vi "Get Fit Results String.vi"(7 "Plot Name":string, 8 "error in (no error)":errorcluster, 9 "Fit Parameters Uncertainties Cluster":variant, 10 "Fit Model":T1, 11 "Fit Parameters Cluster":variant) -> (0 "error out":errorcluster, 3 "Fit Results String":string)   [LabVIEW 2019]
uses:
  Fit Models.ctl
  Gaussian/Gaussian Fit Results v2.ctl
  Lorentzian/Lorentzian Fit Results v2.ctl
  Asymmetric Gaussian/Asymmetric Gaussian Fit Results v2.ctl
  Asymmetric Lorentzian/Asymmetric Lorentzian Fit Results v2.ctl
  Gaussian-Lorentzian/Gaussian-Lorentzian Fit Results v2.ctl
  Lorentzian-Gaussian/Lorentzian-Gaussian Fit Results v2.ctl
  Two Connected Gaussians/Two H-Connected Gaussians Fit Parameters.ctl
  Two Connected Gaussians/Two T-Connected Gaussians Fit Parameters.ctl
  Two Connected Asymmetric Gaussians/Two T-Connected Asymmetric Gaussians Fit Parameters.ctl
  Two Connected Asymmetric Gaussians/Two H-Connected Asymmetric Gaussians Fit Parameters.ctl
  Single Exponential/Single Exponential Fit Parameters v2.ctl
  IRF(X)PSED/IRF(X)PSED Fit Parameters.ctl
  Double Exponential/Double Exponential Fit Parameters v2.ctl
  ACF-CCF/2D ACF/2D Gaussian ACF Fit Results.ctl
  ACF-CCF/2D ACF/2D Gaussian + Blinking ACF Fit Results.ctl
  ACF-CCF/2D ACF/2D Gaussian + Flow ACF Fit Results.ctl
  ACF-CCF/3D ACF/3D Gaussian ACF Fit Results.ctl
  ACF-CCF/3D ACF/3D Gaussian + Blinking ACF Fit Results.ctl
  ACF-CCF/2D ACF/2D Gaussian ACF & 2D Gaussian ACF + Flow Fit Results.ctl
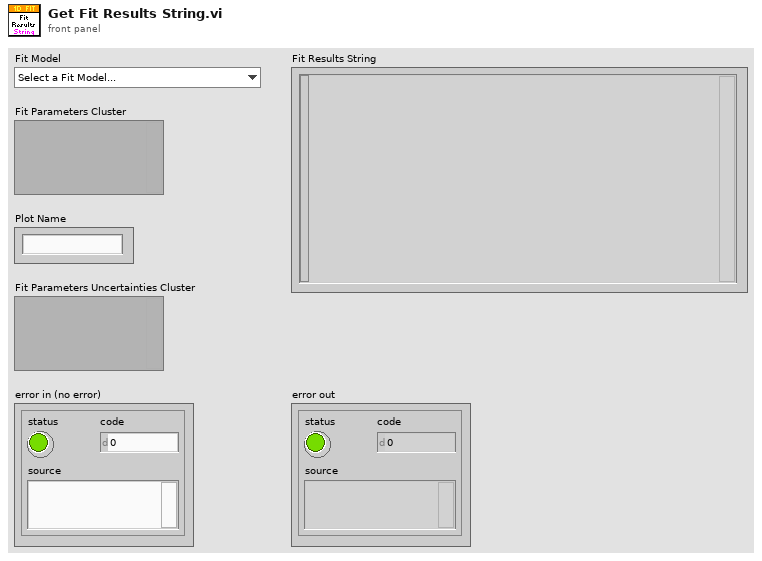
[diagram p1: front panel]
types:
  T1 = typedef "Fit Models.ctl" = enum16{"Select a Fit Model...", "           Single Peak", "Gaussian", "Asymmetric Gaussian", "Lorentzian", "Asymmetric Lorentzian", "Gaussian/Lorentzian", "Lorentzian/Gaussian", "           Double Peak", "Two Gaussians", "Two Asymmetric Gaussians", "Two H-Connected Gaussians", "Two T-Connected Gaussians", "Two H-Connected Asymmetric Gaussians", "Two T-Connected Asymmetric Gaussians", "           Triple Peak", "Three Gaussians", "Three Asymmetric Gaussians", "              Decays", "1-Exponential", "IRF*PSED", "2-Exponentials", "               ACF", "2D Gaussian ACF", "2D Gaussian + Blinking ACF", "2D Gaussian + Flow ACF", "3D Gaussian ACF", "3D Gaussian + Blinking ACF", "             Multiplot", "2D Gaussian ACF & 2D Gaussian + Flow ACF"}
  T2 = typedef "Gaussian Fit Results v2.ctl" = cluster{"Amplitude":dbl, "Peak":dbl, "SDV":dbl, "FWHM":dbl, "Integral":dbl, "RMSE":dbl, "R^2":dbl}
  T3 = typedef "Lorentzian Fit Results v2.ctl" = cluster{"Amplitude":dbl, "Peak":dbl, "FWHM":dbl, "Integral":dbl, "RMSE":dbl, "R^2":dbl}
  T4 = typedef "Asymmetric Gaussian Fit Results v2.ctl" = cluster{"Amplitude":dbl, "Peak":dbl, "SDV-":dbl, "SDV+":dbl, "Mean":dbl, "SDV":dbl, "FWHM":dbl, "Integral":dbl, "RMSE":dbl, "R^2":dbl}
  T5 = typedef "Asymmetric Lorentzian Fit Results v2.ctl" = cluster{"Amplitude":dbl, "Peak":dbl, "FWHM-":dbl, "FWHM+":dbl, "Integral":dbl, "RMSE":dbl, "R^2":dbl}
  T6 = typedef "Gaussian-Lorentzian Fit Results v2.ctl" = cluster{"Amplitude":dbl, "Peak":dbl, "SDV-":dbl, "FWHM+":dbl, "Mean":dbl, "FWHM":dbl, "Integral":dbl, " RMSE":dbl, "R^2":dbl}
  T7 = typedef "Lorentzian-Gaussian Fit Results v2.ctl" = cluster{"Amplitude":dbl, "Peak":dbl, "FWHM-":dbl, "SDV+":dbl, "Mean":dbl, "FWHM":dbl, "Integral":dbl, "RMSE":dbl, "R^2":dbl}
  T8 = typedef "Two H-Connected Gaussians Fit Parameters.ctl" = cluster{"Gaussian Parameters":T2[], "Bridge Amplitude ":dbl}
  T9 = typedef "Two T-Connected Gaussians Fit Parameters.ctl" = cluster{"Gaussian Parameters":T2[], "Bridge Amplitude ":dbl, "Bridge Slope":dbl}
  T10 = typedef "Two T-Connected Asymmetric Gaussians Fit Parameters.ctl" = cluster{"Asymmetric Gaussian Parameters":T4[], "Bridge Amplitude":dbl, "Bridge Slope":dbl}
  T11 = typedef "Two H-Connected Asymmetric Gaussians Fit Parameters.ctl" = cluster{"Asymmetric Gaussian Parameters":T4[], "Bridge Amplitude":dbl}
  T12 = typedef "Single Exponential Fit Parameters v2.ctl" = cluster{"Amplitude":dbl, "Time Constant":dbl, "Baseline":dbl, "Mean":dbl, "SDV":dbl, "FWHM":dbl, "Integral":dbl, "MSE":dbl, "R^2":dbl}
  T13 = typedef "IRF(X)PSED Fit Parameters.ctl" = cluster{"Offset":dbl, "Amplitudes":dbl[], "Time Constants":dbl[], "Baseline":dbl, "Lifetime":dbl, "IRF order":dbl, "Period":dbl, "SDV":dbl, "FWHM":dbl, "Integral":dbl, "MSE":dbl, "R^2":dbl}
  T14 = typedef "Double Exponential Fit Parameters v2.ctl" = cluster{"A1":dbl, "tau1":dbl, "A2":dbl, "tau2":dbl, "Baseline":dbl, "Mean":dbl, "SDV":dbl, "Integral":dbl, "MSE":dbl, "R^2":dbl}
  T15 = typedef "2D Gaussian ACF Fit Results.ctl" = cluster{"Amplitude":dbl, "Diffusion Time":dbl, "RMSE":dbl, "R^2":dbl}
  T16 = typedef "2D Gaussian + Blinking ACF Fit Results.ctl" = cluster{"Amplitude":dbl, "Diffusion Time":dbl, "Blinking Fraction":dbl, "Blinking Time Constant":dbl, "RMSE":dbl, "R^2":dbl}
  T17 = typedef "2D Gaussian + Flow ACF Fit Results.ctl" = cluster{"Amplitude":dbl, "Diffusion Time":dbl, "Translation Time":dbl, "RMSE":dbl, "R^2":dbl}
  T18 = typedef "3D Gaussian ACF Fit Results.ctl" = cluster{"Amplitude":dbl, "Diffusion Time":dbl, "Aspect Ratio":dbl, "RMSE":dbl, "R^2":dbl}
  T19 = typedef "3D Gaussian + Blinking ACF Fit Results.ctl" = cluster{"Amplitude":dbl, "Diffusion Time":dbl, "Aspect Ratio":dbl, "Blinking Fraction":dbl, "Blinking Time Constant":dbl, "RMSE":dbl, "R^2":dbl}
  T20 = typedef "2D Gaussian ACF & 2D Gaussian ACF + Flow Fit Results.ctl" = cluster{"Amplitude 1":dbl, "Diffusion Time":dbl, "Amplitude 2":dbl, "Translation Time":dbl, "RMSE":dbl, "R^2":dbl}
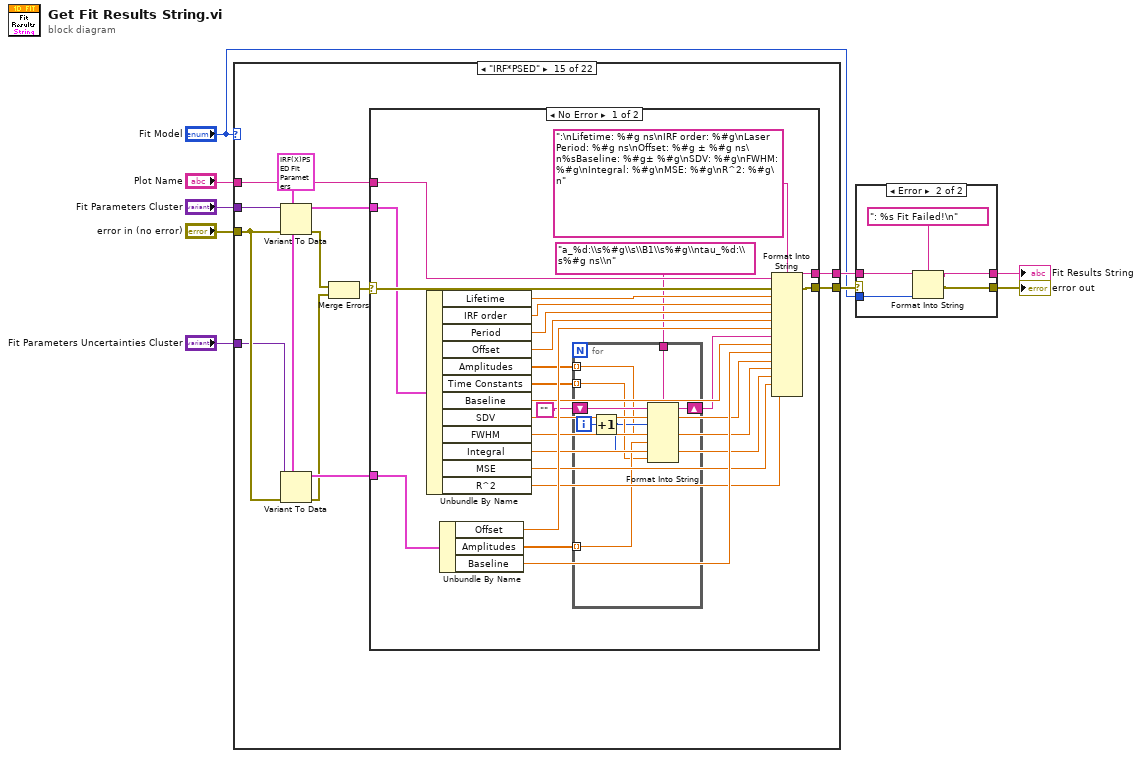
[diagram p0: block diagram]
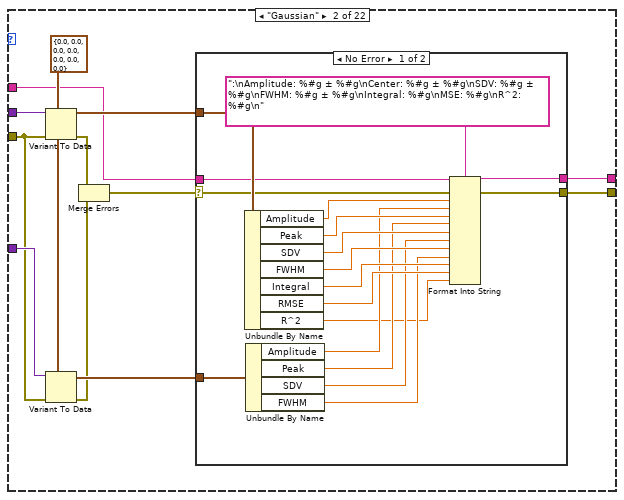
[diagram p4: hidden frame]
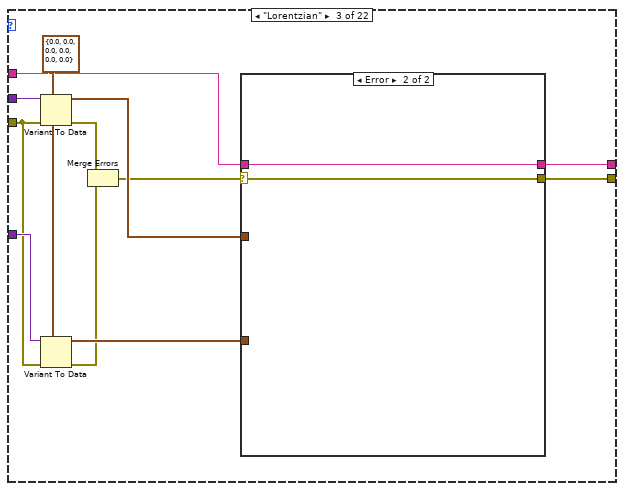
[diagram p6: hidden frame]
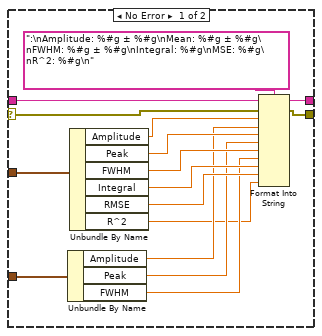
[diagram p7: hidden frame]
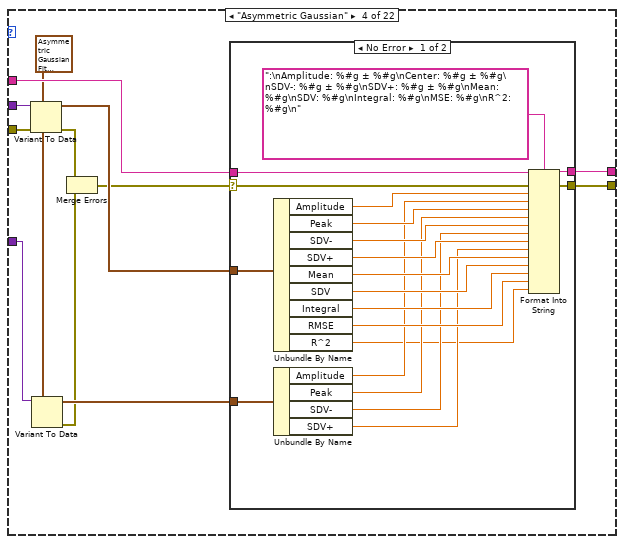
[diagram p8: hidden frame]
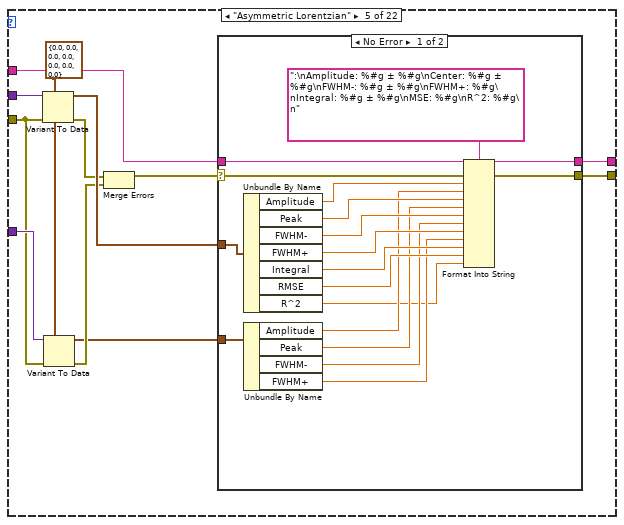
[diagram p10: hidden frame]
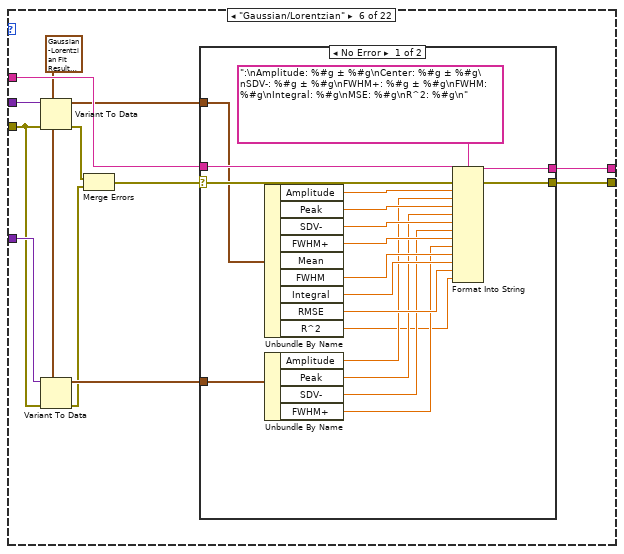
[diagram p12: hidden frame]
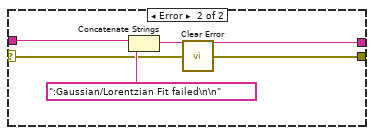
[diagram p13: hidden frame]
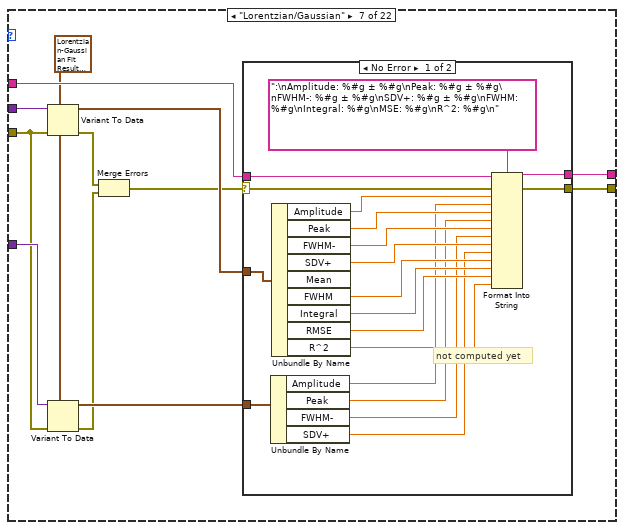
[diagram p14: hidden frame]
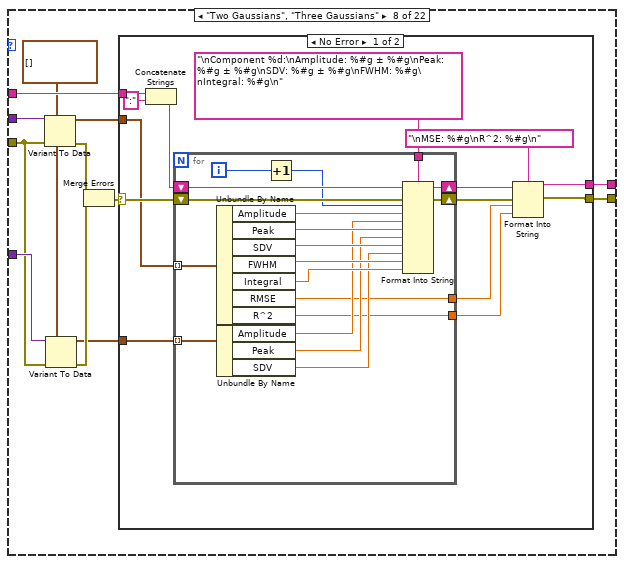
[diagram p16: hidden frame]
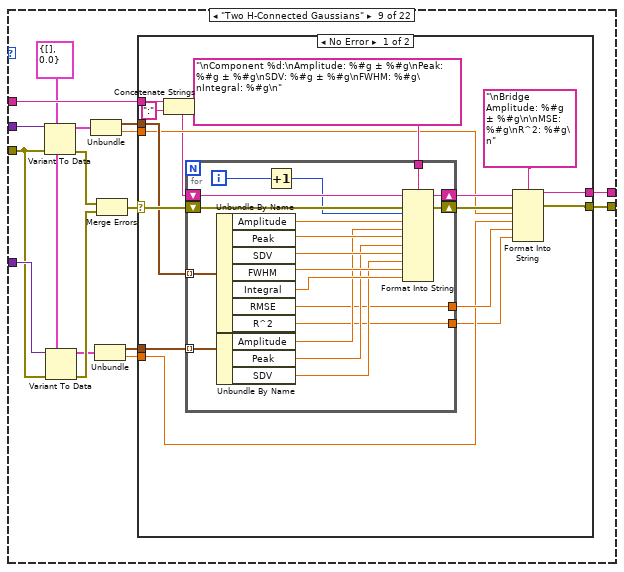
[diagram p18: hidden frame]
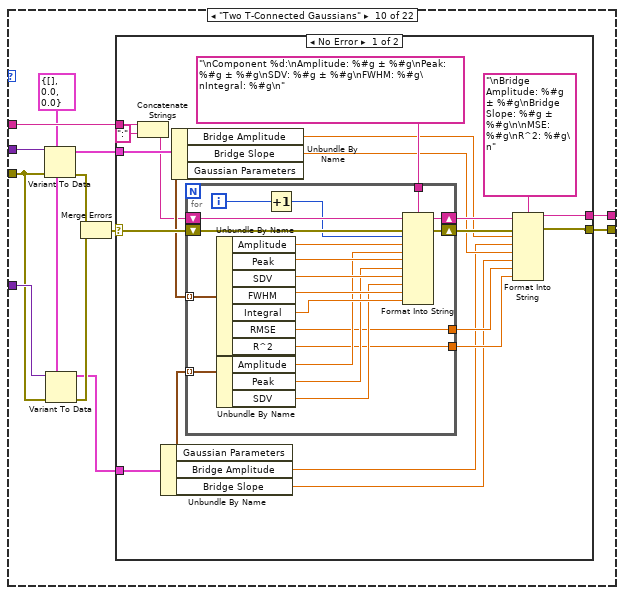
[diagram p20: hidden frame]
diagram:
  n1 = case shown="\"IRF*PSED\"" "Fit Model" {
    tunnel: "error in (no error)" -> [w10 w15 w46 w81 w110 w141 w175 w214 w265 w314 w366 w417 w474 w531 w564 w611 w644 w671 w702 w731 w761 w794]
    tunnel: [w10 w22 w53 w83 w118 w149 w185 w218 w269 w318 w371 w422 w479 w534 w567 w614 w651 w678 w709 w738 w767 w800] -> w5
    tunnel: [_ w21 w54 w84 w117 w150 w186 w219 w270 w319 w372 w423 w480 w535 w568 w615 w650 w677 w708 w737 w766 w799] -> w3
    tunnel: "Fit Parameters Cluster" -> [_ w20 w52 w82 w115 w147 w183 w216 w267 w316 w369 w420 w477 w530 w563 w613 w649 w676 w707 w736 w765 w798]
    tunnel: "Fit Parameters Uncertainties Cluster" -> [_ w18 w50 w76 w111 w142 w179 w215 w266 w315 w367 w418 w475 w524 w557 w612 w647 w674 w705 w734 w763 w796]
    tunnel: "Plot Name" -> [_ w11 w47 w80 w116 w148 w184 w217 w268 w317 w370 w421 w478 w525 w558 w604 w640 w667 w698 w727 w757 w790]
    frame "Select a Fit Model...", Default {
    }
    frame "Gaussian" {
      w17 = T2 {"Amplitude"=0.0, "Peak"=0.0, "SDV"=0.0, "FWHM"=0.0, "Integral"=0.0, "RMSE"=0.0, "R^2"=0.0} ("Gaussian Fit Parameters")
      n2 = Variant To Data(error in=w15, type=w17, Variant=w20) -> (data=w19:T2, error out=w14:errorcluster)
      n3 = Variant To Data(error in=w15, type=w17, Variant=w18) -> (data=w16:T2, error out=w13:errorcluster)
      n4 = Merge Errors(w14, w13) -> (w12:errorcluster)
      n5 = case shown="No Error" w12 {
        selector: w12 -> [w30 w41]
        tunnel: [w40 w41] -> w22
        tunnel: [w39 w42] -> w21
        tunnel: w11 -> [w24 w42]
        tunnel: w19 -> [w37 _]
        tunnel: w16 -> [w29 _]
        frame No Error {
          n6 = Unbundle By Name(w37) -> ("Amplitude"=w36:dbl, "Peak"=w35:dbl, "SDV"=w34:dbl, "FWHM"=w32:dbl, "Integral"=w33:dbl, "RMSE"=w31:dbl, "R^2"=w23:dbl)
          n7 = Unbundle By Name(w29) -> ("Amplitude"=w28:dbl, "Peak"=w27:dbl, "SDV"=w26:dbl, "FWHM"=w25:dbl)
          n8 = Format Into String(format string=":\nAmplitude: %#g ± %#g\nCenter: %#g ± %#g\nSDV: %#g ± %#g\nFWHM: %#g ± %#g\nIntegral: %#g\nMSE: %#g\nR^2: %#g\n", initial string=w24, error in=w30, w36, w28, w35, w27, w34, w26, w32, w25, w33, w31, w23) -> (resulting string=w39:string, error out=w40:errorcluster)
        }
        frame Error {
        }
      }
    }
    frame "Lorentzian" {
      w48 = T3 {"Amplitude"=0.0, "Peak"=0.0, "FWHM"=0.0, "Integral"=0.0, "RMSE"=0.0, "R^2"=0.0} ("Lorentz Fit Parameters")
      n9 = Variant To Data(error in=w46, type=w48, Variant=w52) -> (data=w51:T3, error out=w45:errorcluster)
      n10 = Variant To Data(error in=w46, type=w48, Variant=w50) -> (data=w49:T3, error out=w44:errorcluster)
      n11 = Merge Errors(w45, w44) -> (w43:errorcluster)
      n12 = case shown="Error" w43 {
        selector: w43 -> [w61 w71]
        tunnel: w47 -> [w70 w72]
        tunnel: w51 -> [w69 _]
        tunnel: [w63 w72] -> w54
        tunnel: [w62 w71] -> w53
        tunnel: w49 -> [w59 _]
        frame No Error {
          n13 = Unbundle By Name(w59) -> ("Amplitude"=w58:dbl, "Peak"=w57:dbl, "FWHM"=w56:dbl)
          n14 = Unbundle By Name(w69) -> ("Amplitude"=w67:dbl, "Peak"=w68:dbl, "FWHM"=w66:dbl, "Integral"=w65:dbl, "RMSE"=w64:dbl, "R^2"=w55:dbl)
          n15 = Format Into String(format string=":\nAmplitude: %#g ± %#g\nMean: %#g ± %#g\nFWHM: %#g ± %#g\nIntegral: %#g\nMSE: %#g\nR^2: %#g\n", initial string=w70, error in=w61, w67, w58, w68, w57, w66, w56, w65, w64, w55) -> (resulting string=w63:string, error out=w62:errorcluster)
        }
        frame Error {
        }
      }
    }
    frame "Asymmetric Gaussian" {
      w78 = T4 {"Amplitude"=0.0, "Peak"=0.0, "SDV-"=0.0, "SDV+"=0.0, "Mean"=0.0, "SDV"=0.0, "FWHM"=0.0, "Integral"=0.0, "RMSE"=0.0, "R^2"=0.0} ("Asymmetric Gaussian Fit Parameters")
      n16 = Variant To Data(error in=w81, type=w78, Variant=w82) -> (data=w79:T4, error out=w75:errorcluster)
      n17 = Variant To Data(type=w78, Variant=w76) -> (data=w77:T4, error out=w74:errorcluster)  [unwired: 1 in]
      n18 = Merge Errors(w75, w74) -> (w73:errorcluster)
      n19 = case shown="No Error" w73 {
        selector: w73 -> [w102 w106]
        tunnel: w80 -> [w104 w105]
        tunnel: w79 -> [w91 _]
        tunnel: [w93 w105] -> w84
        tunnel: [w92 w106] -> w83
        tunnel: w77 -> [w90 _]
        frame No Error {
          n20 = Unbundle By Name(w91) -> ("Amplitude"=w98:dbl, "Peak"=w101:dbl, "SDV-"=w100:dbl, "SDV+"=w99:dbl, "Mean"=w97:dbl, "SDV"=w96:dbl, "Integral"=w95:dbl, "RMSE"=w94:dbl, "R^2"=w85:dbl)
          n21 = Unbundle By Name(w90) -> ("Amplitude"=w89:dbl, "Peak"=w88:dbl, "SDV-"=w87:dbl, "SDV+"=w86:dbl)
          n22 = Format Into String(format string=":\nAmplitude: %#g ± %#g\nCenter: %#g ± %#g\nSDV-: %#g ± %#g\nSDV+: %#g ± %#g\nMean: %#g\nSDV: %#g\nIntegral: %#g\nMSE: %#g\nR^2: %#g\n", initial string=w104, error in=w102, w98, w89, w101, w88, w100, w87, w99, w86, w97, w96, w95, w94, w85) -> (resulting string=w93:string, error out=w92:errorcluster)
        }
        frame Error {
        }
      }
    }
    frame "Asymmetric Lorentzian" {
      w112 = T5 {"Amplitude"=0.0, "Peak"=0.0, "FWHM-"=0.0, "FWHM+"=0.0, "Integral"=0.0, "RMSE"=0.0, "R^2"=0.0} ("Asymmetric Lorentz Fit Parameters")
      n23 = Variant To Data(error in=w110, type=w112, Variant=w115) -> (data=w114:T5, error out=w113:errorcluster)
      n24 = Variant To Data(error in=w110, type=w112, Variant=w111) -> (data=w108:T5, error out=w109:errorcluster)
      n25 = Merge Errors(w113, w109) -> (w107:errorcluster)
      n26 = case shown="No Error" w107 {
        selector: w107 -> [w135 w138]
        tunnel: [w128 w138] -> w118
        tunnel: [w127 w137] -> w117
        tunnel: w116 -> [w122 w137]
        tunnel: w114 -> [w121 _]
        tunnel: w108 -> [w120 _]
        frame No Error {
          n27 = Unbundle By Name(w121) -> ("Amplitude"=w131:dbl, "Peak"=w134:dbl, "FWHM-"=w133:dbl, "FWHM+"=w132:dbl, "Integral"=w130:dbl, "RMSE"=w129:dbl, "R^2"=w119:dbl)
          n28 = Unbundle By Name(w120) -> ("Amplitude"=w126:dbl, "Peak"=w125:dbl, "FWHM-"=w124:dbl, "FWHM+"=w123:dbl)
          n29 = Format Into String(format string=":\nAmplitude: %#g ± %#g\nCenter: %#g ± %#g\nFWHM-: %#g ± %#g\nFWHM+: %#g\nIntegral: %#g ± %#g\nMSE: %#g\nR^2: %#g\n", initial string=w122, error in=w135, w131, w126, w134, w125, w133, w124, w132, w123, w130, w129, w119) -> (resulting string=w127:string, error out=w128:errorcluster)
        }
        frame Error {
        }
      }
    }
    frame "Gaussian/Lorentzian" {
      w143 = T6 {"Amplitude"=0.0, "Peak"=0.0, "SDV-"=0.0, "FWHM+"=0.0, "Mean"=0.0, "FWHM"=0.0, "Integral"=0.0, " RMSE"=0.0, "R^2"=0.0} ("Gaussian/Lorentzian Fit Parameters")
      n30 = Variant To Data(error in=w141, type=w143, Variant=w147) -> (data=w144:T6, error out=w146:errorcluster)
      n31 = Variant To Data(error in=w141, type=w143, Variant=w142) -> (data=w140:T6, error out=w139:errorcluster)
      n32 = Merge Errors(w146, w139) -> (w145:errorcluster)
      n33 = case shown="No Error" w145 {
        selector: w145 -> [w167 w171]
        tunnel: w148 -> [w169 w173]
        tunnel: [w159 w172] -> w150
        tunnel: [w158 w170] -> w149
        tunnel: w144 -> [w153 _]
        tunnel: w140 -> [w152 _]
        frame No Error {
          n34 = Unbundle By Name(w153) -> ("Amplitude"=w165:dbl, "Peak"=w166:dbl, "SDV-"=w164:dbl, "FWHM+"=w163:dbl, "FWHM"=w162:dbl, "Integral"=w161:dbl, "RMSE"=w160:dbl, "R^2"=w151:dbl)  [unwired: 1 out]
          n35 = Unbundle By Name(w152) -> ("Amplitude"=w157:dbl, "Peak"=w156:dbl, "SDV-"=w155:dbl, "FWHM+"=w154:dbl)
          n36 = Format Into String(format string=":\nAmplitude: %#g ± %#g\nCenter: %#g ± %#g\nSDV-: %#g ± %#g\nFWHM+: %#g ± %#g\nFWHM: %#g\nIntegral: %#g\nMSE: %#g\nR^2: %#g\n", initial string=w169, error in=w167, w165, w157, w166, w156, w164, w155, w163, w154, w162, w161, w160, w151) -> (resulting string=w159:string, error out=w158:errorcluster)
        }
        frame Error {
          n37 = Concatenate Strings(w173, ":Gaussian/Lorentzian Fit failed\n\n" ("format string")) -> (w172:string)
          n38 = call "Clear Error.vi"("Error In"=w171) -> ("no Error Out"=w170:errorcluster)  [unwired: 8 in]
        }
      }
    }
    frame "Lorentzian/Gaussian" {
      w178 = T7 {"Amplitude"=0.0, "Peak"=0.0, "FWHM-"=0.0, "SDV+"=0.0, "Mean"=0.0, "FWHM"=0.0, "Integral"=0.0, "RMSE"=0.0, "R^2"=0.0} ("Lorentzian/Gaussian Fit Parameters")
      n39 = Variant To Data(error in=w175, type=w178, Variant=w183) -> (data=w182:T7, error out=w181:errorcluster)
      n40 = Variant To Data(error in=w175, type=w178, Variant=w179) -> (data=w177:T7, error out=w176:errorcluster)
      n41 = Merge Errors(w181, w176) -> (w180:errorcluster)
      n42 = case shown="No Error" w180 {
        selector: w180 -> [w204 w207]
        tunnel: [w196 w206] -> w186
        tunnel: [w195 w207] -> w185
        tunnel: w184 -> [w190 w206]
        tunnel: w182 -> [w189 _]
        tunnel: w177 -> [w188 _]
        frame No Error {
          # "not computed yet"
          n43 = Unbundle By Name(w188) -> ("Amplitude"=w194:dbl, "Peak"=w193:dbl, "FWHM-"=w192:dbl, "SDV+"=w191:dbl)
          n44 = Unbundle By Name(w189) -> ("Amplitude"=w202:dbl, "Peak"=w203:dbl, "FWHM-"=w200:dbl, "SDV+"=w201:dbl, "FWHM"=w199:dbl, "Integral"=w198:dbl, "RMSE"=w197:dbl, "R^2"=w187:dbl)  [unwired: 1 out]
          n45 = Format Into String(format string=":\nAmplitude: %#g ± %#g\nPeak: %#g ± %#g\nFWHM-: %#g ± %#g\nSDV+: %#g ± %#g\nFWHM: %#g\nIntegral: %#g\nMSE: %#g\nR^2: %#g\n", initial string=w190, error in=w204, w202, w194, w203, w193, w200, w192, w201, w191, w199, w198, w197, w187) -> (resulting string=w196:string, error out=w195:errorcluster)
        }
        frame Error {
        }
      }
    }
    frame "Two Gaussians", "Three Gaussians" {
      w208 = T2[] [] ("Array")
      n46 = Variant To Data(error in=w214, type=w208, Variant=w216) -> (data=w210:T2[], error out=w213:errorcluster)
      n47 = Variant To Data(error in=w214, type=w208, Variant=w215) -> (data=w209:T2[], error out=w212:errorcluster)
      n48 = Merge Errors(w213, w212) -> (w211:errorcluster)
      n49 = case shown="No Error" w211 {
        selector: w211 -> [w232 w254]
        tunnel: [w227 w253] -> w219
        tunnel: [w225 w254] -> w218
        tunnel: w217 -> [w230 w253]
        tunnel: w210 -> [w229 _]
        tunnel: w209 -> [w228 _]
        frame No Error {
          n50 = Concatenate Strings(w230, ":" ("string")) -> (w221:string)
          n51 = for {
            tunnel: "\nComponent %d:\nAmplitude: %#g ± %#g\nPeak: %#g ± %#g\nSDV: %#g ± %#g\nFWHM: %#g\nIntegral: %#g\n" ("format string") -> [w252]
            shift-right: [w245] -> w226
            shift-left: w232 -> [w251]
            shift-right: [w246] -> w231
            shift-left: w221 -> [w244]
            tunnel: w229 -> [w237] mode=indexing
            tunnel: w228 -> [w236] mode=indexing
            tunnel: [w235] -> w223
            tunnel: [w234] -> w222
            i -> [w239]
            n52 = Unbundle By Name(w237) -> ("Amplitude"=w240:dbl, "Peak"=w250:dbl, "SDV"=w249:dbl, "FWHM"=w248:dbl, "Integral"=w247:dbl, "RMSE"=w235:dbl, "R^2"=w234:dbl)
            n53 = Unbundle By Name(w236) -> ("Amplitude"=w243:dbl, "Peak"=w242:dbl, "SDV"=w241:dbl)
            n54 = Increment(x=w239) -> (x+1=w238:i32)
            n55 = Format Into String(format string=w252, initial string=w244, error in=w251, w238, w240, w243, w250, w242, w249, w241, w248, w247) -> (resulting string=w246:string, error out=w245:errorcluster)
          }
          n56 = Format Into String(format string="\nMSE: %#g\nR^2: %#g\n", initial string=w231, error in=w226, w223, w222) -> (resulting string=w227:string, error out=w225:errorcluster)
        }
        frame Error {
        }
      }
    }
    frame "Two H-Connected Gaussians" {
      w259 = T8 {"Gaussian Parameters"=[], "Bridge Amplitude "=0.0} ("Bridged Gaussians Parameters")
      n57 = Variant To Data(error in=w265, type=w259, Variant=w267) -> (data=w261:T8, error out=w264:errorcluster)
      n58 = Variant To Data(error in=w265, type=w259, Variant=w266) -> (data=w260:T8, error out=w263:errorcluster)
      n59 = Unbundle(w261) -> ("Gaussian Parameters"=w258:T2[], "Bridge Amplitude"=w256:dbl)
      n60 = Unbundle(w260) -> ("Gaussian Parameters"=w257:T2[], "Bridge Amplitude"=w255:dbl)
      n61 = Merge Errors(w264, w263) -> (w262:errorcluster)
      n62 = case shown="No Error" w262 {
        selector: w262 -> [w285 w307]
        tunnel: [w281 w306] -> w270
        tunnel: [w279 w307] -> w269
        tunnel: w268 -> [w272 w306]
        tunnel: w258 -> [w283 _]
        tunnel: w257 -> [w282 _]
        tunnel: w256 -> [w275 _]
        tunnel: w255 -> [w276 _]
        frame No Error {
          n63 = Concatenate Strings(w272, ":" ("string")) -> (w271:string)
          n64 = for {
            tunnel: "\nComponent %d:\nAmplitude: %#g ± %#g\nPeak: %#g ± %#g\nSDV: %#g ± %#g\nFWHM: %#g\nIntegral: %#g\n" ("format string") -> [w305]
            shift-right: [w298] -> w280
            shift-left: w285 -> [w304]
            shift-right: [w299] -> w284
            shift-left: w271 -> [w297]
            tunnel: w283 -> [w290] mode=indexing
            tunnel: w282 -> [w289] mode=indexing
            tunnel: [w288] -> w277
            tunnel: [w287] -> w274
            i -> [w292]
            n65 = Unbundle By Name(w290) -> ("Amplitude"=w293:dbl, "Peak"=w303:dbl, "SDV"=w302:dbl, "FWHM"=w301:dbl, "Integral"=w300:dbl, "RMSE"=w288:dbl, "R^2"=w287:dbl)
            n66 = Unbundle By Name(w289) -> ("Amplitude"=w296:dbl, "Peak"=w295:dbl, "SDV"=w294:dbl)
            n67 = Increment(x=w292) -> (x+1=w291:i32)
            n68 = Format Into String(format string=w305, initial string=w297, error in=w304, w291, w293, w296, w303, w295, w302, w294, w301, w300) -> (resulting string=w299:string, error out=w298:errorcluster)
          }
          n69 = Format Into String(format string="\nBridge Amplitude: %#g ± %#g\n\nMSE: %#g\nR^2: %#g\n", initial string=w284, error in=w280, w275, w276, w277, w274) -> (resulting string=w281:string, error out=w279:errorcluster)
        }
        frame Error {
        }
      }
    }
    frame "Two T-Connected Gaussians" {
      w310 = T9 {"Gaussian Parameters"=[], "Bridge Amplitude "=0.0, "Bridge Slope"=0.0} ("Bridged Gaussians Parameters")
      n70 = Variant To Data(error in=w314, type=w310, Variant=w316) -> (data=w309:T9, error out=w313:errorcluster)
      n71 = Variant To Data(error in=w314, type=w310, Variant=w315) -> (data=w308:T9, error out=w312:errorcluster)
      n72 = Merge Errors(w313, w312) -> (w311:errorcluster)
      n73 = case shown="No Error" w311 {
        selector: w311 -> [w338 w360]
        tunnel: [w336 w359] -> w319
        tunnel: [w334 w360] -> w318
        tunnel: w317 -> [w321 w359]
        tunnel: w309 -> [w330 _]
        tunnel: w308 -> [w326 _]
        frame No Error {
          n74 = Concatenate Strings(w321, ":" ("string")) -> (w320:string)
          n75 = Unbundle By Name(w326) -> ("Gaussian Parameters"=w325:T2[], "Bridge Amplitude"=w324:dbl, "Bridge Slope"=w323:dbl)
          n76 = Unbundle By Name(w330) -> ("Bridge Amplitude"=w328:dbl, "Bridge Slope"=w327:dbl, "Gaussian Parameters"=w329:T2[])
          n77 = for {
            tunnel: "\nComponent %d:\nAmplitude: %#g ± %#g\nPeak: %#g ± %#g\nSDV: %#g ± %#g\nFWHM: %#g\nIntegral: %#g\n" ("format string") -> [w358]
            shift-right: [w351] -> w335
            shift-left: w338 -> [w357]
            shift-right: [w352] -> w337
            shift-left: w320 -> [w350]
            tunnel: w329 -> [w343] mode=indexing
            tunnel: w325 -> [w342] mode=indexing
            tunnel: [w341] -> w332
            tunnel: [w340] -> w331
            i -> [w345]
            n78 = Unbundle By Name(w343) -> ("Amplitude"=w346:dbl, "Peak"=w356:dbl, "SDV"=w355:dbl, "FWHM"=w354:dbl, "Integral"=w353:dbl, "RMSE"=w341:dbl, "R^2"=w340:dbl)
            n79 = Unbundle By Name(w342) -> ("Amplitude"=w349:dbl, "Peak"=w348:dbl, "SDV"=w347:dbl)
            n80 = Increment(x=w345) -> (x+1=w344:i32)
            n81 = Format Into String(format string=w358, initial string=w350, error in=w357, w344, w346, w349, w356, w348, w355, w347, w354, w353) -> (resulting string=w352:string, error out=w351:errorcluster)
          }
          n82 = Format Into String(format string="\nBridge Amplitude: %#g ± %#g\nBridge Slope: %#g ± %#g\n\nMSE: %#g\nR^2: %#g\n", initial string=w337, error in=w335, w328, w324, w327, w323, w332, w331) -> (resulting string=w336:string, error out=w334:errorcluster)
        }
        frame Error {
        }
      }
    }
    frame "Two Asymmetric Gaussians", "Three Asymmetric Gaussians" {
      w365 = T4[] [] ("Array")
      n83 = Variant To Data(error in=w366, type=w365, Variant=w367) -> (data=w361:T4[], error out=w364:errorcluster)
      n84 = Variant To Data(error in=w366, type=w365, Variant=w369) -> (data=w362:T4[], error out=w368:errorcluster)
      n85 = Merge Errors(w368, w364) -> (w363:errorcluster)
      n86 = case shown="No Error" w363 {
        selector: w363 -> [w385 w410]
        tunnel: w370 -> [w386 w411]
        tunnel: [w378 w411] -> w372
        tunnel: [w376 w410] -> w371
        tunnel: w362 -> [w384 _]
        tunnel: w361 -> [w383 _]
        frame No Error {
          n87 = Concatenate Strings(w386, ":" ("string")) -> (w381:string)
          n88 = for {
            shift-right: [w399] -> w379
            shift-left: w381 -> [w402]
            shift-right: [w400] -> w377
            shift-left: w385 -> [w401]
            tunnel: w384 -> [w398] mode=indexing
            tunnel: w383 -> [w397] mode=indexing
            tunnel: "\nComponent %d:\nAmplitude: %#g ± %#g\nCenter: %#g ± %#g\nSDV-: %#g ± %#g\nSDV+: %#g ± %#g\nMean: %#g\nSDV: %#g\nFWHM: %#g\nIntegral: %#g\n" ("format string") -> [w396]
            tunnel: [w388] -> w375
            tunnel: [w387] -> w373
            i -> [w394]
            n89 = Unbundle By Name(w398) -> ("Amplitude"=w395:dbl, "Peak"=w409:dbl, "SDV-"=w408:dbl, "SDV+"=w407:dbl, "Mean"=w406:dbl, "SDV"=w405:dbl, "FWHM"=w404:dbl, "Integral"=w403:dbl, "RMSE"=w388:dbl, "R^2"=w387:dbl)
            n90 = Unbundle By Name(w397) -> ("Amplitude"=w392:dbl, "Peak"=w391:dbl, "SDV-"=w390:dbl, "SDV+"=w389:dbl)
            n91 = Increment(x=w394) -> (x+1=w393:i32)
            n92 = Format Into String(format string=w396, initial string=w402, error in=w401, w393, w395, w392, w409, w391, w408, w390, w407, w389, w406, w405, w404, w403) -> (resulting string=w399:string, error out=w400:errorcluster)
          }
          n93 = Format Into String(format string="\nMSE: %#g\nR^2: %#g\n", initial string=w379, error in=w377, w375, w373) -> (resulting string=w378:string, error out=w376:errorcluster)
        }
        frame Error {
        }
      }
    }
    frame "Two T-Connected Asymmetric Gaussians" {
      w412 = T10 {"Asymmetric Gaussian Parameters"=[], "Bridge Amplitude"=0.0, "Bridge Slope"=0.0} ("Two T-Connected Asymmetric Gaussian Parameters")
      n94 = Variant To Data(error in=w417, type=w412, Variant=w418) -> (data=w413:T10, error out=w416:errorcluster)
      n95 = Variant To Data(error in=w417, type=w412, Variant=w420) -> (data=w414:T10, error out=w419:errorcluster)
      n96 = Merge Errors(w419, w416) -> (w415:errorcluster)
      n97 = case shown="No Error" w415 {
        selector: w415 -> [w442 w467]
        tunnel: w421 -> [w443 w468]
        tunnel: [w436 w468] -> w423
        tunnel: [w435 w467] -> w422
        tunnel: w414 -> [w441 _]
        tunnel: w413 -> [w427 _]
        frame No Error {
          n98 = Unbundle By Name(w441) -> ("Bridge Amplitude"=w431:dbl, "Bridge Slope"=w430:dbl, "Asymmetric Gaussian Parameters"=w428:T4[])
          n99 = Concatenate Strings(w443, ":" ("string")) -> (w439:string)
          n100 = Unbundle By Name(w427) -> ("Asymmetric Gaussian Parameters"=w426:T4[], "Bridge Amplitude"=w425:dbl, "Bridge Slope"=w424:dbl)
          n101 = for {
            shift-right: [w456] -> w437
            shift-left: w439 -> [w459]
            shift-right: [w457] -> w434
            shift-left: w442 -> [w458]
            tunnel: w428 -> [w455] mode=indexing
            tunnel: w426 -> [w454] mode=indexing
            tunnel: "\nComponent %d:\nAmplitude: %#g ± %#g\nCenter: %#g ± %#g\nSDV-: %#g ± %#g\nSDV+: %#g ± %#g\nMean: %#g\nSDV: %#g\nFWHM: %#g\nIntegral: %#g\n" ("format string") -> [w453]
            tunnel: [w445] -> w432
            tunnel: [w444] -> w429
            i -> [w451]
            n102 = Unbundle By Name(w455) -> ("Amplitude"=w452:dbl, "Peak"=w466:dbl, "SDV-"=w465:dbl, "SDV+"=w464:dbl, "Mean"=w463:dbl, "SDV"=w462:dbl, "FWHM"=w461:dbl, "Integral"=w460:dbl, "RMSE"=w445:dbl, "R^2"=w444:dbl)
            n103 = Unbundle By Name(w454) -> ("Amplitude"=w449:dbl, "Peak"=w448:dbl, "SDV-"=w447:dbl, "SDV+"=w446:dbl)
            n104 = Increment(x=w451) -> (x+1=w450:i32)
            n105 = Format Into String(format string=w453, initial string=w459, error in=w458, w450, w452, w449, w466, w448, w465, w447, w464, w446, w463, w462, w461, w460) -> (resulting string=w456:string, error out=w457:errorcluster)
          }
          n106 = Format Into String(format string="\nBridge Amplitude: %#g ± %#g\nBridge Slope: %#g ± %#g\n\nMSE: %#g\nR^2: %#g\n", initial string=w437, error in=w434, w431, w425, w430, w424, w432, w429) -> (resulting string=w436:string, error out=w435:errorcluster)
        }
        frame Error {
        }
      }
    }
    frame "Two H-Connected Asymmetric Gaussians" {
      w471 = T11 {"Asymmetric Gaussian Parameters"=[], "Bridge Amplitude"=0.0} ("output cluster")
      n107 = Variant To Data(error in=w474, type=w471, Variant=w475) -> (data=w469:T11, error out=w473:errorcluster)
      n108 = Variant To Data(error in=w474, type=w471, Variant=w477) -> (data=w470:T11, error out=w476:errorcluster)
      n109 = Merge Errors(w476, w473) -> (w472:errorcluster)
      n110 = case shown="No Error" w472 {
        selector: w472 -> [w497 w522]
        tunnel: w478 -> [w498 w523]
        tunnel: [w492 w523] -> w480
        tunnel: [w490 w522] -> w479
        tunnel: w470 -> [w485 _]
        tunnel: w469 -> [w484 _]
        frame No Error {
          n111 = Unbundle(w484) -> ("Asymmetric Gaussian Parameters"=w483:T4[], "Bridge Amplitude"=w482:dbl)
          n112 = Unbundle(w485) -> ("Asymmetric Gaussian Parameters"=w487:T4[], "Bridge Amplitude"=w486:dbl)
          n113 = Concatenate Strings(w498, ":" ("string")) -> (w495:string)
          n114 = for {
            shift-right: [w511] -> w493
            shift-left: w495 -> [w514]
            shift-right: [w512] -> w491
            shift-left: w497 -> [w513]
            tunnel: w487 -> [w510] mode=indexing
            tunnel: w483 -> [w509] mode=indexing
            tunnel: "\nComponent %d:\nAmplitude: %#g ± %#g\nCenter: %#g ± %#g\nSDV-: %#g ± %#g\nSDV+: %#g ± %#g\nMean: %#g\nSDV: %#g\nFWHM: %#g\nIntegral: %#g\n" ("format string") -> [w508]
            tunnel: [w500] -> w488
            tunnel: [w499] -> w481
            i -> [w506]
            n115 = Unbundle By Name(w510) -> ("Amplitude"=w507:dbl, "Peak"=w521:dbl, "SDV-"=w520:dbl, "SDV+"=w519:dbl, "Mean"=w518:dbl, "SDV"=w517:dbl, "FWHM"=w516:dbl, "Integral"=w515:dbl, "RMSE"=w500:dbl, "R^2"=w499:dbl)
            n116 = Unbundle By Name(w509) -> ("Amplitude"=w504:dbl, "Peak"=w503:dbl, "SDV-"=w502:dbl, "SDV+"=w501:dbl)
            n117 = Increment(x=w506) -> (x+1=w505:i32)
            n118 = Format Into String(format string=w508, initial string=w514, error in=w513, w505, w507, w504, w521, w503, w520, w502, w519, w501, w518, w517, w516, w515) -> (resulting string=w511:string, error out=w512:errorcluster)
          }
          n119 = Format Into String(format string="\nBridge Amplitude: %#g ± %#g\n\nMSE: %#g\nR^2: %#g\n", initial string=w493, error in=w491, w486, w482, w488, w481) -> (resulting string=w492:string, error out=w490:errorcluster)
        }
        frame Error {
        }
      }
    }
    frame "1-Exponential" {
      w532 = T12 {"Amplitude"=0.0, "Time Constant"=0.0, "Baseline"=0.0, "Mean"=0.0, "SDV"=0.0, "FWHM"=0.0, "Integral"=0.0, "MSE"=0.0, "R^2"=0.0} ("Single Exponential Fit Parameters")
      n120 = Variant To Data(error in=w531, type=w532, Variant=w530) -> (data=w533:T12, error out=w528:errorcluster)
      n121 = Variant To Data(error in=w531, type=w532, Variant=w524) -> (data=w529:T12, error out=w527:errorcluster)
      n122 = Merge Errors(w528, w527) -> (w526:errorcluster)
      n123 = case shown="No Error" w526 {
        selector: w526 -> [w553 w556]
        tunnel: [w545 w555] -> w535
        tunnel: [w544 w556] -> w534
        tunnel: w533 -> [w541 _]
        tunnel: w529 -> [w540 _]
        tunnel: w525 -> [w539 w555]
        frame No Error {
          n124 = Unbundle By Name(w541) -> ("Amplitude"=w551:dbl, "Time Constant"=w552:dbl, "Baseline"=w537:dbl, "Mean"=w550:dbl, "SDV"=w549:dbl, "FWHM"=w548:dbl, "Integral"=w547:dbl, "MSE"=w546:dbl, "R^2"=w538:dbl)
          n125 = Unbundle By Name(w540) -> ("Amplitude"=w543:dbl, "Time Constant"=w542:dbl, "Baseline"=w536:dbl)
          n126 = Format Into String(format string=":\nAmplitude: %#g ± %#g\nTime Constant: %#g ± %#g\nBaseline: %#g ± %#g\nMean: %#g\nSDV: %#g\nFWHM: %#g\nIntegral: %#g\nMSE: %#g\nR^2: %#g\n", initial string=w539, error in=w553, w551, w543, w552, w542, w537, w536, w550, w549, w548, w547, w546, w538) -> (resulting string=w545:string, error out=w544:errorcluster)
        }
        frame Error {
        }
      }
    }
    frame "IRF*PSED" {
      w565 = T13 {"Offset"=0.0, "Amplitudes"=[], "Time Constants"=[], "Baseline"=0.0, "Lifetime"=0.0, "IRF order"=0.0, "Period"=0.0, "SDV"=0.0, "FWHM"=0.0, "Integral"=0.0, "MSE"=0.0, "R^2"=0.0} ("IRF*PSED Fit Parameters")
      n127 = Variant To Data(error in=w564, type=w565, Variant=w563) -> (data=w566:T13, error out=w561:errorcluster)
      n128 = Variant To Data(error in=w564, type=w565, Variant=w557) -> (data=w562:T13, error out=w560:errorcluster)
      n129 = Merge Errors(w561, w560) -> (w559:errorcluster)
      n130 = case shown="No Error" w559 {
        selector: w559 -> [w592 w603]
        tunnel: [w590 w602] -> w568
        tunnel: [w589 w603] -> w567
        tunnel: w566 -> [w588 _]
        tunnel: w562 -> [w587 _]
        tunnel: w558 -> [w586 w602]
        frame No Error {
          n131 = Unbundle By Name(w588) -> ("Lifetime"=w591:dbl, "IRF order"=w585:dbl, "Period"=w584:dbl, "Offset"=w583:dbl, "Amplitudes"=w581:dbl[], "Time Constants"=w580:dbl[], "Baseline"=w578:dbl, "SDV"=w576:dbl, "FWHM"=w575:dbl, "Integral"=w574:dbl, "MSE"=w573:dbl, "R^2"=w572:dbl)
          n132 = Unbundle By Name(w587) -> ("Offset"=w582:dbl, "Amplitudes"=w579:dbl[], "Baseline"=w577:dbl)
          n133 = for {
            tunnel: w581 -> [w594] mode=indexing
            tunnel: w580 -> [w597] mode=indexing
            tunnel: w579 -> [w598] mode=indexing
            tunnel: "a_%d:\\s%#g\\s\\B1\\s%#g\\ntau_%d:\\s%#g ns\\n" -> [w601]
            shift-right: [w599] -> w570
            shift-left: "" -> [w600]
            i -> [w596]
            n134 = Increment(x=w596) -> (x+1=w595:i32)
            n135 = Format Into String(format string=w601, initial string=w600, w595, w594, w598, w595, w597) -> (resulting string=w599:string)  [unwired: 1 in, 1 out]
          }
          n136 = Format Into String(format string=":\nLifetime: %#g ns\nIRF order: %#g\nLaser Period: %#g ns\nOffset: %#g ± %#g ns\n%sBaseline: %#g± %#g\nSDV: %#g\nFWHM: %#g\nIntegral: %#g\nMSE: %#g\nR^2: %#g\n", initial string=w586, error in=w592, w591, w585, w584, w583, w582, w570, w578, w577, w576, w575, w574, w573, w572) -> (resulting string=w590:string, error out=w589:errorcluster)
        }
        frame Error {
        }
      }
    }
    frame "2-Exponentials" {
      w608 = T14 {"A1"=0.0, "tau1"=0.0, "A2"=0.0, "tau2"=0.0, "Baseline"=0.0, "Mean"=0.0, "SDV"=0.0, "Integral"=0.0, "MSE"=0.0, "R^2"=0.0} ("Double Exponential Fit Parameters")
      n137 = Variant To Data(error in=w611, type=w608, Variant=w613) -> (data=w610:T14, error out=w607:errorcluster)
      n138 = Variant To Data(error in=w611, type=w608, Variant=w612) -> (data=w609:T14, error out=w606:errorcluster)
      n139 = Merge Errors(w607, w606) -> (w605:errorcluster)
      n140 = case shown="No Error" w605 {
        selector: w605 -> [w636 w639]
        tunnel: [w627 w638] -> w615
        tunnel: [w626 w639] -> w614
        tunnel: w610 -> [w621 _]
        tunnel: w609 -> [w620 _]
        tunnel: w604 -> [w619 w638]
        frame No Error {
          n141 = Unbundle By Name(w620) -> ("A1"=w625:dbl, "tau1"=w624:dbl, "A2"=w623:dbl, "tau2"=w622:dbl, "Baseline"=w616:dbl)
          n142 = Unbundle By Name(w621) -> ("A1"=w634:dbl, "tau1"=w635:dbl, "A2"=w629:dbl, "tau2"=w628:dbl, "Baseline"=w617:dbl, "Mean"=w633:dbl, "SDV"=w632:dbl, "Integral"=w631:dbl, "MSE"=w630:dbl, "R^2"=w618:dbl)
          n143 = Format Into String(format string=":\nA1: %#g ± %#g\nTau 1: %#g ± %#g\nA2: %#g ± %#g\nTau 2: %#g ± %#g\nBaseline: %#g ± %#g\nMean: %#g\nSDV: %#g\nIntegral: %#g\nMSE: %#g\nR^2: %#g\n", initial string=w619, error in=w636, w634, w625, w635, w624, w629, w623, w628, w622, w617, w616, w633, w632, w631, w630, w618) -> (resulting string=w627:string, error out=w626:errorcluster)
        }
        frame Error {
        }
      }
    }
    frame "2D Gaussian ACF" {
      w646 = T15 {"Amplitude"=0.0, "Diffusion Time"=0.0, "RMSE"=0.0, "R^2"=0.0} ("2D ACF Fit Parameters")
      n144 = Variant To Data(error in=w644, type=w646, Variant=w649) -> (data=w648:T15, error out=w643:errorcluster)
      n145 = Variant To Data(error in=w644, type=w646, Variant=w647) -> (data=w645:T15, error out=w642:errorcluster)
      n146 = Merge Errors(w643, w642) -> (w641:errorcluster)
      n147 = case shown="No Error" w641 {
        selector: w641 -> [w658 w665]
        tunnel: [w664 w665] -> w651
        tunnel: [w663 w666] -> w650
        tunnel: w640 -> [w654 w666]
        tunnel: w648 -> [w661 _]
        tunnel: w645 -> [w657 _]
        frame No Error {
          n148 = Unbundle By Name(w661) -> ("Amplitude"=w660:dbl, "Diffusion Time"=w652:dbl, "RMSE"=w659:dbl, "R^2"=w653:dbl)
          n149 = Unbundle By Name(w657) -> ("Amplitude"=w656:dbl, "Diffusion Time"=w655:dbl)
          n150 = Format Into String(format string=":\nAmplitude: %#g ± %#g\nDiffusion Time: %#g ± %#g\nMSE: %#g\nR^2: %#g\n", initial string=w654, error in=w658, w660, w656, w652, w655, w659, w653) -> (resulting string=w663:string, error out=w664:errorcluster)
        }
        frame Error {
        }
      }
    }
    frame "2D Gaussian + Blinking ACF" {
      w673 = T16 {"Amplitude"=0.0, "Diffusion Time"=0.0, "Blinking Fraction"=0.0, "Blinking Time Constant"=0.0, "RMSE"=0.0, "R^2"=0.0} ("2D Gaussian + Blinking ACF Fit Parameters")
      n151 = Variant To Data(error in=w671, type=w673, Variant=w676) -> (data=w675:T16, error out=w670:errorcluster)
      n152 = Variant To Data(error in=w671, type=w673, Variant=w674) -> (data=w672:T16, error out=w669:errorcluster)
      n153 = Merge Errors(w670, w669) -> (w668:errorcluster)
      n154 = case shown="No Error" w668 {
        selector: w668 -> [w689 w696]
        tunnel: [w695 w696] -> w678
        tunnel: [w694 w697] -> w677
        tunnel: w667 -> [w685 w697]
        tunnel: w675 -> [w692 _]
        tunnel: w672 -> [w688 _]
        frame No Error {
          n155 = Unbundle By Name(w692) -> ("Amplitude"=w691:dbl, "Diffusion Time"=w683:dbl, "Blinking Fraction"=w682:dbl, "Blinking Time Constant"=w681:dbl, "RMSE"=w690:dbl, "R^2"=w684:dbl)
          n156 = Unbundle By Name(w688) -> ("Amplitude"=w687:dbl, "Diffusion Time"=w686:dbl, "Blinking Fraction"=w680:dbl, "Blinking Time Constant"=w679:dbl)
          n157 = Format Into String(format string=":\nAmplitude: %#g ± %#g\nDiffusion Time: %#g ± %#g\nBlinking Fraction: %#g ± %#g\nBlinking Time Constant: %#g ± %#g\nMSE: %#g\nR^2: %#g\n", initial string=w685, error in=w689, w691, w687, w683, w686, w682, w680, w681, w679, w690, w684) -> (resulting string=w694:string, error out=w695:errorcluster)
        }
        frame Error {
        }
      }
    }
    frame "2D Gaussian + Flow ACF" {
      w704 = T17 {"Amplitude"=0.0, "Diffusion Time"=0.0, "Translation Time"=0.0, "RMSE"=0.0, "R^2"=0.0} ("2D Gaussian + Blinking ACF Fit Parameters")
      n158 = Variant To Data(error in=w702, type=w704, Variant=w707) -> (data=w706:T17, error out=w701:errorcluster)
      n159 = Variant To Data(error in=w702, type=w704, Variant=w705) -> (data=w703:T17, error out=w700:errorcluster)
      n160 = Merge Errors(w701, w700) -> (w699:errorcluster)
      n161 = case shown="No Error" w699 {
        selector: w699 -> [w718 w725]
        tunnel: [w724 w725] -> w709
        tunnel: [w723 w726] -> w708
        tunnel: w698 -> [w714 w726]
        tunnel: w706 -> [w721 _]
        tunnel: w703 -> [w717 _]
        frame No Error {
          n162 = Unbundle By Name(w721) -> ("Amplitude"=w720:dbl, "Diffusion Time"=w712:dbl, "Translation Time"=w711:dbl, "RMSE"=w719:dbl, "R^2"=w713:dbl)
          n163 = Unbundle By Name(w717) -> ("Amplitude"=w716:dbl, "Diffusion Time"=w715:dbl, "Translation Time"=w710:dbl)
          n164 = Format Into String(format string=":\nAmplitude: %#g ± %#g\nDiffusion Time: %#g ± %#g\nTranslation Time Constant: %#g ± %#g\nMSE: %#g\nR^2: %#g\n", initial string=w714, error in=w718, w720, w716, w712, w715, w711, w710, w719, w713) -> (resulting string=w723:string, error out=w724:errorcluster)
        }
        frame Error {
        }
      }
    }
    frame "3D Gaussian ACF" {
      w733 = T18 {"Amplitude"=0.0, "Diffusion Time"=0.0, "Aspect Ratio"=0.0, "RMSE"=0.0, "R^2"=0.0} ("3D ACF Fit Parameters")
      n165 = Variant To Data(error in=w731, type=w733, Variant=w736) -> (data=w735:T18, error out=w730:errorcluster)
      n166 = Variant To Data(error in=w731, type=w733, Variant=w734) -> (data=w732:T18, error out=w729:errorcluster)
      n167 = Merge Errors(w730, w729) -> (w728:errorcluster)
      n168 = case shown="No Error" w728 {
        selector: w728 -> [w747 w754]
        tunnel: [w753 w754] -> w738
        tunnel: [w752 w755] -> w737
        tunnel: w727 -> [w744 w755]
        tunnel: w735 -> [w750 _]
        tunnel: w732 -> [w746 _]
        frame No Error {
          n169 = Unbundle By Name(w750) -> ("Amplitude"=w749:dbl, "Diffusion Time"=w742:dbl, "Aspect Ratio"=w740:dbl, "RMSE"=w748:dbl, "R^2"=w743:dbl)
          n170 = Unbundle By Name(w746) -> ("Amplitude"=w745:dbl, "Diffusion Time"=w741:dbl, "Aspect Ratio"=w739:dbl)
          n171 = Format Into String(format string=":\nAmplitude: %#g ± %#g\nDiffusion Time: %#g ± %#g\nAspect Ratio: %#g ± %#g\nMSE: %#g\nR^2: %#g\n", initial string=w744, error in=w747, w749, w745, w742, w741, w740, w739, w748, w743) -> (resulting string=w752:string, error out=w753:errorcluster)
        }
        frame Error {
        }
      }
    }
    frame "3D Gaussian + Blinking ACF" {
      w756 = T19 {"Amplitude"=0.0, "Diffusion Time"=0.0, "Aspect Ratio"=0.0, "Blinking Fraction"=0.0, "Blinking Time Constant"=0.0, "RMSE"=0.0, "R^2"=0.0} ("2D Gaussian + Blinking ACF Fit Parameters")
      n172 = Variant To Data(error in=w761, type=w756, Variant=w765) -> (data=w764:T19, error out=w760:errorcluster)
      n173 = Variant To Data(error in=w761, type=w756, Variant=w763) -> (data=w762:T19, error out=w759:errorcluster)
      n174 = Merge Errors(w760, w759) -> (w758:errorcluster)
      n175 = case shown="No Error" w758 {
        selector: w758 -> [w780 w787]
        tunnel: [w786 w787] -> w767
        tunnel: [w785 w788] -> w766
        tunnel: w757 -> [w776 w788]
        tunnel: w764 -> [w783 _]
        tunnel: w762 -> [w779 _]
        frame No Error {
          n176 = Unbundle By Name(w783) -> ("Amplitude"=w782:dbl, "Diffusion Time"=w774:dbl, "Aspect Ratio"=w769:dbl, "Blinking Fraction"=w773:dbl, "Blinking Time Constant"=w772:dbl, "RMSE"=w781:dbl, "R^2"=w775:dbl)
          n177 = Unbundle By Name(w779) -> ("Amplitude"=w778:dbl, "Diffusion Time"=w777:dbl, "Aspect Ratio"=w768:dbl, "Blinking Fraction"=w771:dbl, "Blinking Time Constant"=w770:dbl)
          n178 = Format Into String(format string=":\nAmplitude: %#g ± %#g\nDiffusion Time: %#g ± %#g\nAspect Ratio: %#g ± %#g\nBlinking Fraction: %#g ± %#g\nBlinking Time Constant: %#g ± %#g\nMSE: %#g\nR^2: %#g\n", initial string=w776, error in=w780, w782, w778, w774, w777, w769, w768, w773, w771, w772, w770, w781, w775) -> (resulting string=w785:string, error out=w786:errorcluster)
        }
        frame Error {
        }
      }
    }
    frame "2D Gaussian ACF & 2D Gaussian + Flow ACF" {
      w789 = T20 {"Amplitude 1"=0.0, "Diffusion Time"=0.0, "Amplitude 2"=0.0, "Translation Time"=0.0, "RMSE"=0.0, "R^2"=0.0} ("2D Gaussian ACF & ACF + Flow Fit Parameters")
      n179 = Variant To Data(error in=w794, type=w789, Variant=w798) -> (data=w797:T20, error out=w793:errorcluster)
      n180 = Variant To Data(error in=w794, type=w789, Variant=w796) -> (data=w795:T20, error out=w792:errorcluster)
      n181 = Merge Errors(w793, w792) -> (w791:errorcluster)
      n182 = case shown="No Error" w791 {
        selector: w791 -> [w811 w818]
        tunnel: [w817 w818] -> w800
        tunnel: [w816 w819] -> w799
        tunnel: w790 -> [w807 w819]
        tunnel: w797 -> [w814 _]
        tunnel: w795 -> [w810 _]
        frame No Error {
          n183 = Unbundle By Name(w814) -> ("Amplitude 1"=w813:dbl, "Diffusion Time"=w805:dbl, "Amplitude 2"=w802:dbl, "Translation Time"=w804:dbl, "RMSE"=w812:dbl, "R^2"=w806:dbl)
          n184 = Unbundle By Name(w810) -> ("Amplitude 1"=w809:dbl, "Diffusion Time"=w808:dbl, "Amplitude 2"=w801:dbl, "Translation Time"=w803:dbl)
          n185 = Format Into String(format string=":\nAmplitude 1: %#g ± %#g\nDiffusion Time: %#g ± %#g\nAmplitude 2: %#g ± %#g\nTranslation Time Constant: %#g ± %#g\nMSE: %#g\nR^2: %#g\n", initial string=w807, error in=w811, w813, w809, w805, w808, w802, w801, w804, w803, w812, w806) -> (resulting string=w816:string, error out=w817:errorcluster)
        }
        frame Error {
        }
      }
    }
  }
  n186 = case shown="Error" w5 {
    selector: w5 -> [w821 _]
    tunnel: [w821 w823] -> w4
    tunnel: w3 -> [w820 w825]
    tunnel: "Fit Model" -> [_ w824]
    tunnel: [w820 w822] -> w2
    frame No Error {
    }
    frame Error {
      n187 = Format Into String(format string=": %s Fit Failed!\n", initial string=w825, w824) -> (resulting string=w822:string, error out=w823:errorcluster)  [unwired: 1 in]
    }
  }
  "error out" <- w4
  "Fit Results String" <- w2
